vi "Global Value.vi"() -> ()   [LabVIEW 2014]
panel:
  in  "Delay_ms":u32=1000
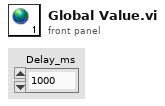
[diagram p1: front panel]
diagram:
